vi "Strain_configuration_REV0_2019_02_25.vi"(8 "error in":errorcluster) -> (0 "error out":errorcluster, 3 "task out":refnum<k21>)   [LabVIEW 2017]
uses:
  <vilib>/DAQmx/create/channels.llb/DAQmx Create Channel (AI-Strain-Strain Gage).vi
  <resource>/objmgr/daqmx.rc
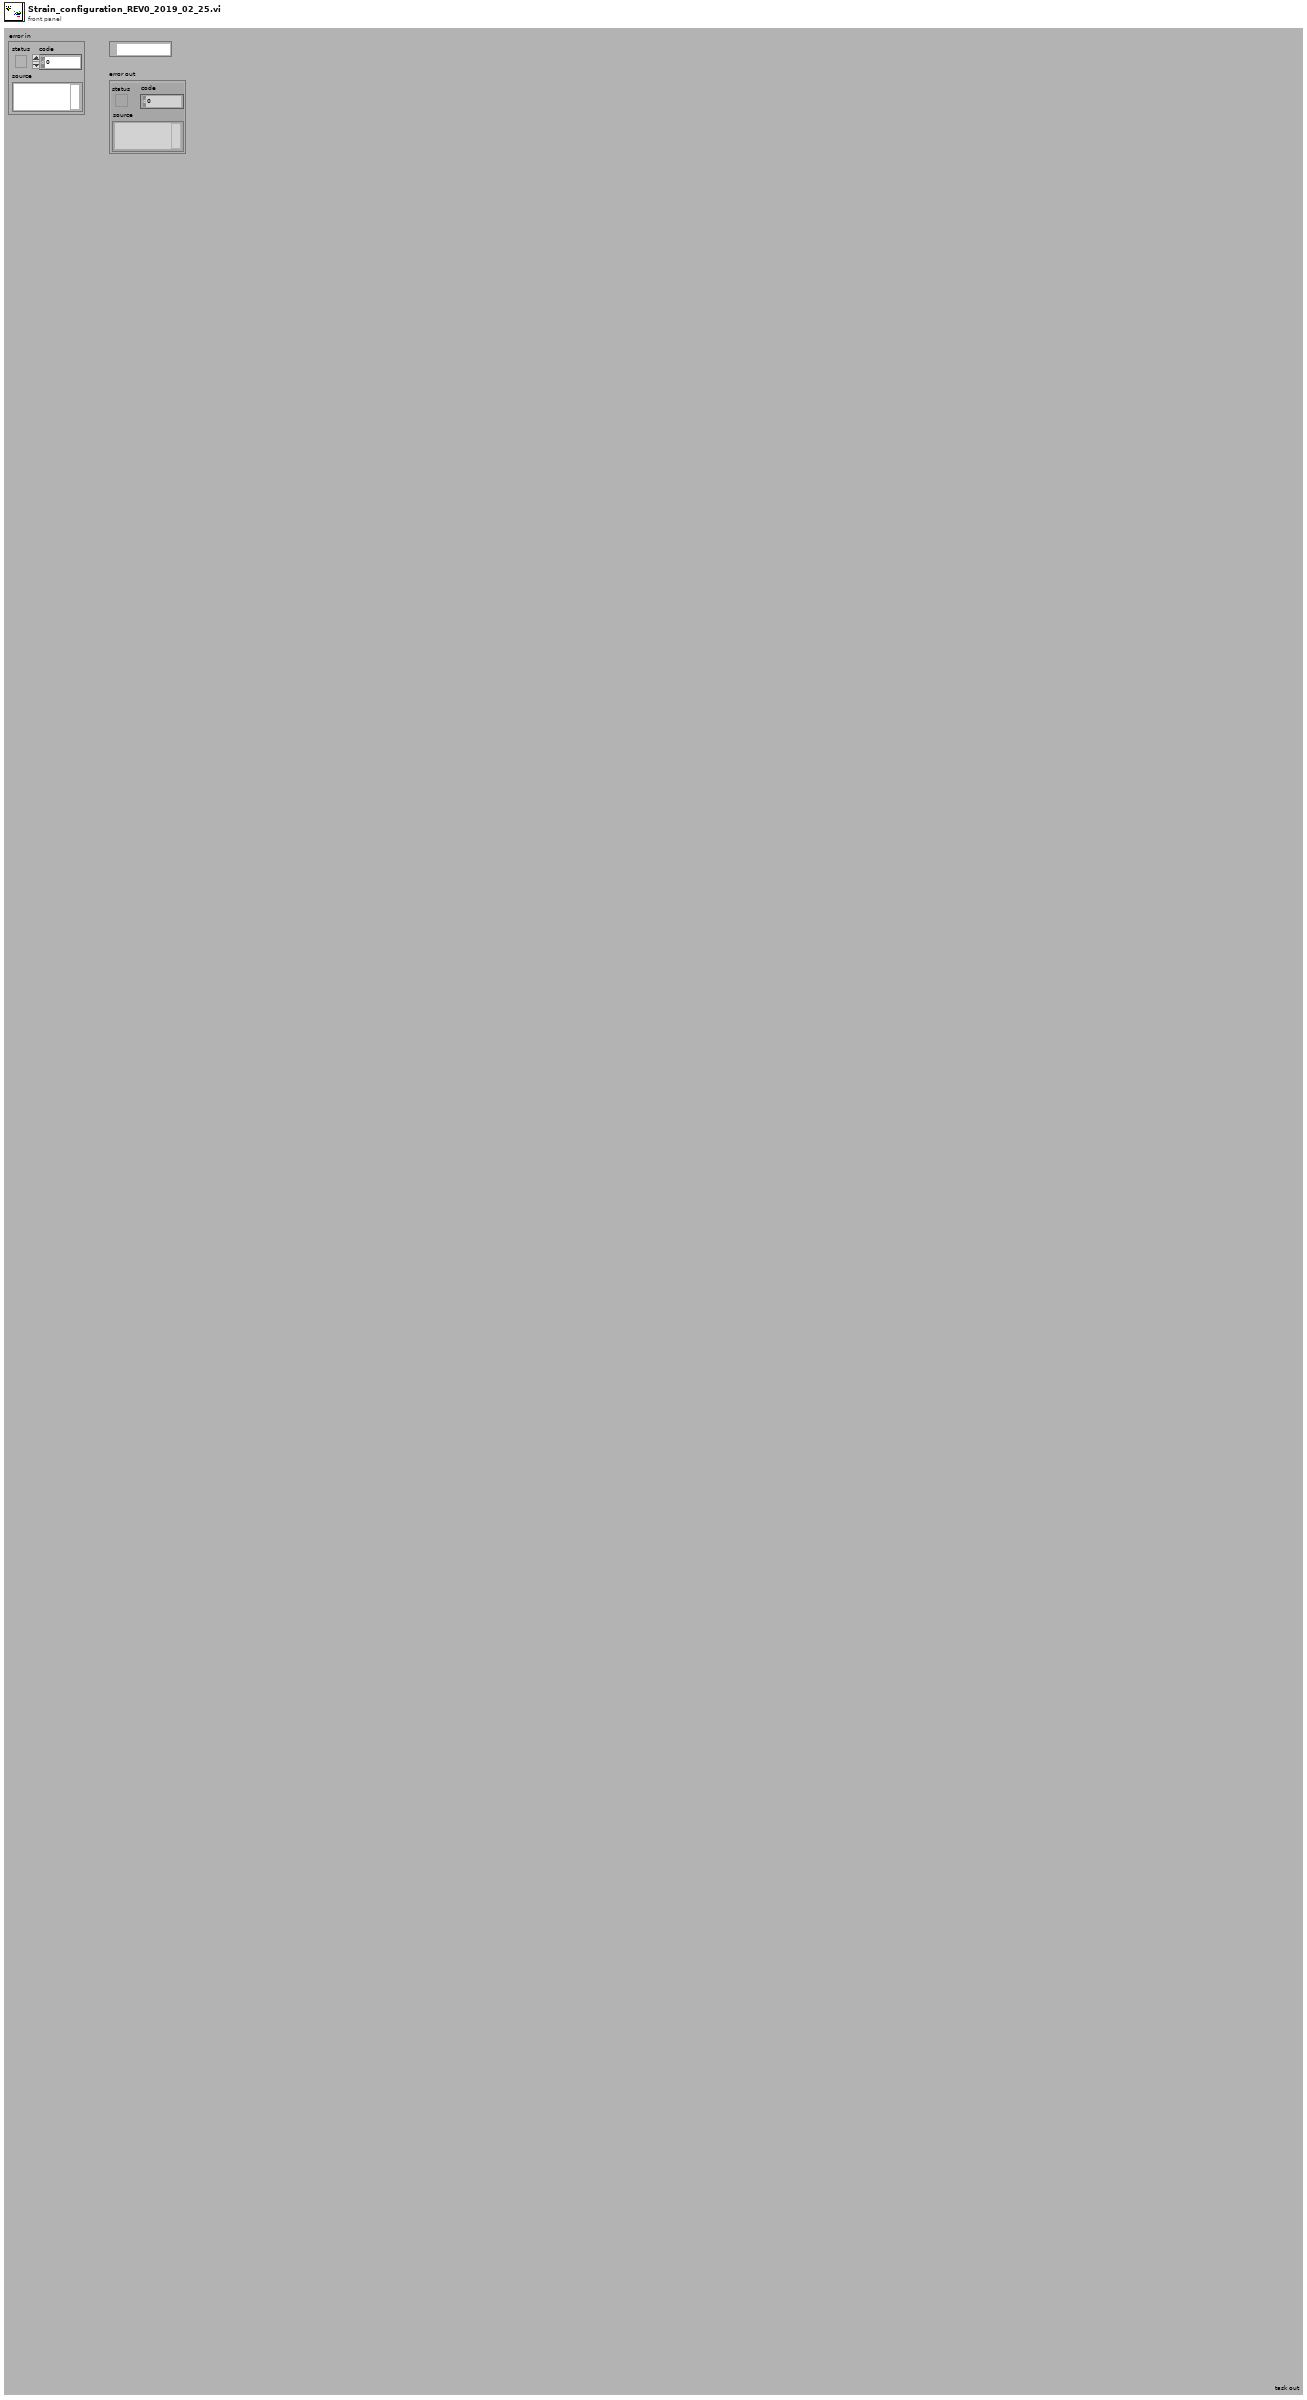
[diagram p1: front panel]
types:
  T1 = cluster{"strain configuration":i32, "lead resistance":dbl, "initial bridge voltage":dbl, "excitation source":i32, "excitation value":dbl}
  T2 = cluster{"gage factor":dbl, "nominal gage resistance":dbl, "poisson ratio":dbl}
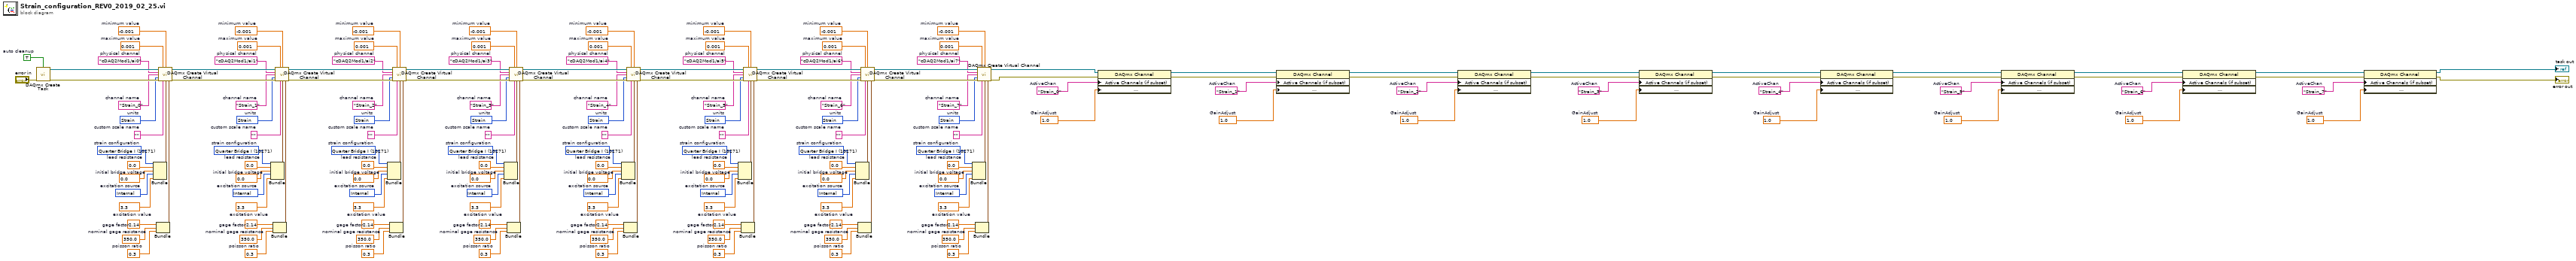
[diagram p0: block diagram]
diagram:
  w3 = 1.0  # GainAdjust
  w5 = "Strain_7"  # ActiveChan
  w6 = 1.0  # GainAdjust
  w9 = "Strain_6"  # ActiveChan
  w10 = 1.0  # GainAdjust
  w13 = "Strain_5"  # ActiveChan
  w14 = 1.0  # GainAdjust
  w17 = "Strain_4"  # ActiveChan
  w18 = 1.0  # GainAdjust
  w21 = "Strain_3"  # ActiveChan
  w22 = 1.0  # GainAdjust
  w25 = "Strain_2"  # ActiveChan
  w26 = 1.0  # GainAdjust
  w29 = "Strain_1"  # ActiveChan
  w30 = 1.0  # GainAdjust
  w33 = "Strain_0"  # ActiveChan
  w38 = 0.0  # lead resistance
  w41 = 0.3  # poisson ratio
  w37 = 0.0  # initial bridge voltage
  w42 = 350.0  # nominal gage resistance
  w40 = 2.14  # gage factor
  w35 = 3.3  # excitation value
  w36 = 10200 items=["Internal"=10200, "External"=10167, "None"=10230]  # excitation source
  w39 = 10271 items=["Full Bridge I"=10183, "Full Bridge II"=10184, "Full Bridge III"=10185, "Half Bridge I"=10188, "Half Bridge II"=10189, "Quarter Bridge I"=10271, "Quarter Bridge II"=10272]  # strain configuration
  w44 = 10299 items=["Strain"=10299, "From Custom Scale"=10065]  # units
  w45 = "Strain_7"  # channel name
  w47 = ""  # custom scale name
  w48 = -0.001  # minimum value
  w49 = 0.001  # maximum value
  w50 = "cDAQ2Mod1/ai7"  # physical channel
  w56 = 0.0  # lead resistance
  w59 = 0.3  # poisson ratio
  w55 = 0.0  # initial bridge voltage
  w60 = 350.0  # nominal gage resistance
  w58 = 2.14  # gage factor
  w53 = 3.3  # excitation value
  w54 = 10200 items=["Internal"=10200, "External"=10167, "None"=10230]  # excitation source
  w57 = 10271 items=["Full Bridge I"=10183, "Full Bridge II"=10184, "Full Bridge III"=10185, "Half Bridge I"=10188, "Half Bridge II"=10189, "Quarter Bridge I"=10271, "Quarter Bridge II"=10272]  # strain configuration
  w62 = 10299 items=["Strain"=10299, "From Custom Scale"=10065]  # units
  w63 = "Strain_6"  # channel name
  w65 = ""  # custom scale name
  w66 = -0.001  # minimum value
  w67 = 0.001  # maximum value
  w68 = "cDAQ2Mod1/ai6"  # physical channel
  w74 = 0.0  # lead resistance
  w77 = 0.3  # poisson ratio
  w73 = 0.0  # initial bridge voltage
  w78 = 350.0  # nominal gage resistance
  w76 = 2.14  # gage factor
  w71 = 3.3  # excitation value
  w72 = 10200 items=["Internal"=10200, "External"=10167, "None"=10230]  # excitation source
  w75 = 10271 items=["Full Bridge I"=10183, "Full Bridge II"=10184, "Full Bridge III"=10185, "Half Bridge I"=10188, "Half Bridge II"=10189, "Quarter Bridge I"=10271, "Quarter Bridge II"=10272]  # strain configuration
  w80 = 10299 items=["Strain"=10299, "From Custom Scale"=10065]  # units
  w81 = "Strain_5"  # channel name
  w83 = ""  # custom scale name
  w84 = -0.001  # minimum value
  w85 = 0.001  # maximum value
  w86 = "cDAQ2Mod1/ai5"  # physical channel
  w92 = 0.0  # lead resistance
  w95 = 0.3  # poisson ratio
  w91 = 0.0  # initial bridge voltage
  w96 = 350.0  # nominal gage resistance
  w94 = 2.14  # gage factor
  w89 = 3.3  # excitation value
  w90 = 10200 items=["Internal"=10200, "External"=10167, "None"=10230]  # excitation source
  w93 = 10271 items=["Full Bridge I"=10183, "Full Bridge II"=10184, "Full Bridge III"=10185, "Half Bridge I"=10188, "Half Bridge II"=10189, "Quarter Bridge I"=10271, "Quarter Bridge II"=10272]  # strain configuration
  w98 = 10299 items=["Strain"=10299, "From Custom Scale"=10065]  # units
  w99 = "Strain_4"  # channel name
  w101 = ""  # custom scale name
  w102 = -0.001  # minimum value
  w103 = 0.001  # maximum value
  w104 = "cDAQ2Mod1/ai4"  # physical channel
  w110 = 0.0  # lead resistance
  w113 = 0.3  # poisson ratio
  w109 = 0.0  # initial bridge voltage
  w114 = 350.0  # nominal gage resistance
  w112 = 2.14  # gage factor
  w107 = 3.3  # excitation value
  w108 = 10200 items=["Internal"=10200, "External"=10167, "None"=10230]  # excitation source
  w111 = 10271 items=["Full Bridge I"=10183, "Full Bridge II"=10184, "Full Bridge III"=10185, "Half Bridge I"=10188, "Half Bridge II"=10189, "Quarter Bridge I"=10271, "Quarter Bridge II"=10272]  # strain configuration
  w116 = 10299 items=["Strain"=10299, "From Custom Scale"=10065]  # units
  w117 = "Strain_3"  # channel name
  w119 = ""  # custom scale name
  w120 = -0.001  # minimum value
  w121 = 0.001  # maximum value
  w122 = "cDAQ2Mod1/ai3"  # physical channel
  w128 = 0.0  # lead resistance
  w131 = 0.3  # poisson ratio
  w127 = 0.0  # initial bridge voltage
  w132 = 350.0  # nominal gage resistance
  w130 = 2.14  # gage factor
  w125 = 3.3  # excitation value
  w126 = 10200 items=["Internal"=10200, "External"=10167, "None"=10230]  # excitation source
  w129 = 10271 items=["Full Bridge I"=10183, "Full Bridge II"=10184, "Full Bridge III"=10185, "Half Bridge I"=10188, "Half Bridge II"=10189, "Quarter Bridge I"=10271, "Quarter Bridge II"=10272]  # strain configuration
  w134 = 10299 items=["Strain"=10299, "From Custom Scale"=10065]  # units
  w135 = "Strain_2"  # channel name
  w137 = ""  # custom scale name
  w138 = -0.001  # minimum value
  w139 = 0.001  # maximum value
  w140 = "cDAQ2Mod1/ai2"  # physical channel
  w146 = 0.0  # lead resistance
  w149 = 0.3  # poisson ratio
  w145 = 0.0  # initial bridge voltage
  w150 = 350.0  # nominal gage resistance
  w148 = 2.14  # gage factor
  w143 = 3.3  # excitation value
  w144 = 10200 items=["Internal"=10200, "External"=10167, "None"=10230]  # excitation source
  w147 = 10271 items=["Full Bridge I"=10183, "Full Bridge II"=10184, "Full Bridge III"=10185, "Half Bridge I"=10188, "Half Bridge II"=10189, "Quarter Bridge I"=10271, "Quarter Bridge II"=10272]  # strain configuration
  w152 = 10299 items=["Strain"=10299, "From Custom Scale"=10065]  # units
  w153 = "Strain_1"  # channel name
  w155 = ""  # custom scale name
  w156 = -0.001  # minimum value
  w157 = 0.001  # maximum value
  w158 = "cDAQ2Mod1/ai1"  # physical channel
  w164 = 0.0  # lead resistance
  w167 = 0.3  # poisson ratio
  w163 = 0.0  # initial bridge voltage
  w168 = 350.0  # nominal gage resistance
  w166 = 2.14  # gage factor
  w161 = 3.3  # excitation value
  w162 = 10200 items=["Internal"=10200, "External"=10167, "None"=10230]  # excitation source
  w165 = 10271 items=["Full Bridge I"=10183, "Full Bridge II"=10184, "Full Bridge III"=10185, "Half Bridge I"=10188, "Half Bridge II"=10189, "Quarter Bridge I"=10271, "Quarter Bridge II"=10272]  # strain configuration
  w170 = 10299 items=["Strain"=10299, "From Custom Scale"=10065]  # units
  w171 = "Strain_0"  # channel name
  w173 = ""  # custom scale name
  w174 = -0.001  # minimum value
  w175 = 0.001  # maximum value
  w176 = "cDAQ2Mod1/ai0"  # physical channel
  w178 = TRUE  # auto cleanup
  n1 = call <vilib>:"DAQmx Create Task.vi"("auto cleanup"=w178, "error in"="error in") -> ("task out"=w177:refnum<k21>, "error out"=w179:errorcluster)  [unwired: 12 in]
  n2 = Bundle("strain configuration"=w165, "lead resistance"=w164, "initial bridge voltage"=w163, "excitation source"=w162, "excitation value"=w161) -> (w160:T1)  [unwired: 1 in]
  n3 = Bundle("gage factor"=w166, "nominal gage resistance"=w168, "poisson ratio"=w167) -> (w169:T2)  [unwired: 1 in]
  n4 = call-poly <vilib>:"DAQmx Create Virtual Channel.vi"("task in"=w177, "maximum value"=w175, "minimum value"=w174, "physical channels"=w176, "name to assign"=w171, "units"=w170, "error in"=w179, "custom scale name"=w173, "bridge information"=w160, "strain gage information"=w169) -> ("task out"=w159:refnum<k21>, "error out"=w172:errorcluster)  [unwired: 4 in]
  n5 = Bundle("strain configuration"=w147, "lead resistance"=w146, "initial bridge voltage"=w145, "excitation source"=w144, "excitation value"=w143) -> (w142:T1)  [unwired: 1 in]
  n6 = Bundle("gage factor"=w148, "nominal gage resistance"=w150, "poisson ratio"=w149) -> (w151:T2)  [unwired: 1 in]
  n7 = call-poly <vilib>:"DAQmx Create Virtual Channel.vi"("task in"=w159, "maximum value"=w157, "minimum value"=w156, "physical channels"=w158, "name to assign"=w153, "units"=w152, "error in"=w172, "custom scale name"=w155, "bridge information"=w142, "strain gage information"=w151) -> ("task out"=w141:refnum<k21>, "error out"=w154:errorcluster)  [unwired: 4 in]
  n8 = Bundle("strain configuration"=w129, "lead resistance"=w128, "initial bridge voltage"=w127, "excitation source"=w126, "excitation value"=w125) -> (w124:T1)  [unwired: 1 in]
  n9 = Bundle("gage factor"=w130, "nominal gage resistance"=w132, "poisson ratio"=w131) -> (w133:T2)  [unwired: 1 in]
  n10 = call-poly <vilib>:"DAQmx Create Virtual Channel.vi"("task in"=w141, "maximum value"=w139, "minimum value"=w138, "physical channels"=w140, "name to assign"=w135, "units"=w134, "error in"=w154, "custom scale name"=w137, "bridge information"=w124, "strain gage information"=w133) -> ("task out"=w123:refnum<k21>, "error out"=w136:errorcluster)  [unwired: 4 in]
  n11 = Bundle("strain configuration"=w111, "lead resistance"=w110, "initial bridge voltage"=w109, "excitation source"=w108, "excitation value"=w107) -> (w106:T1)  [unwired: 1 in]
  n12 = Bundle("gage factor"=w112, "nominal gage resistance"=w114, "poisson ratio"=w113) -> (w115:T2)  [unwired: 1 in]
  n13 = call-poly <vilib>:"DAQmx Create Virtual Channel.vi"("task in"=w123, "maximum value"=w121, "minimum value"=w120, "physical channels"=w122, "name to assign"=w117, "units"=w116, "error in"=w136, "custom scale name"=w119, "bridge information"=w106, "strain gage information"=w115) -> ("task out"=w105:refnum<k21>, "error out"=w118:errorcluster)  [unwired: 4 in]
  n14 = Bundle("strain configuration"=w93, "lead resistance"=w92, "initial bridge voltage"=w91, "excitation source"=w90, "excitation value"=w89) -> (w88:T1)  [unwired: 1 in]
  n15 = Bundle("gage factor"=w94, "nominal gage resistance"=w96, "poisson ratio"=w95) -> (w97:T2)  [unwired: 1 in]
  n16 = call-poly <vilib>:"DAQmx Create Virtual Channel.vi"("task in"=w105, "maximum value"=w103, "minimum value"=w102, "physical channels"=w104, "name to assign"=w99, "units"=w98, "error in"=w118, "custom scale name"=w101, "bridge information"=w88, "strain gage information"=w97) -> ("task out"=w87:refnum<k21>, "error out"=w100:errorcluster)  [unwired: 4 in]
  n17 = Bundle("strain configuration"=w75, "lead resistance"=w74, "initial bridge voltage"=w73, "excitation source"=w72, "excitation value"=w71) -> (w70:T1)  [unwired: 1 in]
  n18 = Bundle("gage factor"=w76, "nominal gage resistance"=w78, "poisson ratio"=w77) -> (w79:T2)  [unwired: 1 in]
  n19 = call-poly <vilib>:"DAQmx Create Virtual Channel.vi"("task in"=w87, "maximum value"=w85, "minimum value"=w84, "physical channels"=w86, "name to assign"=w81, "units"=w80, "error in"=w100, "custom scale name"=w83, "bridge information"=w70, "strain gage information"=w79) -> ("task out"=w69:refnum<k21>, "error out"=w82:errorcluster)  [unwired: 4 in]
  n20 = Bundle("strain configuration"=w57, "lead resistance"=w56, "initial bridge voltage"=w55, "excitation source"=w54, "excitation value"=w53) -> (w52:T1)  [unwired: 1 in]
  n21 = Bundle("gage factor"=w58, "nominal gage resistance"=w60, "poisson ratio"=w59) -> (w61:T2)  [unwired: 1 in]
  n22 = call-poly <vilib>:"DAQmx Create Virtual Channel.vi"("task in"=w69, "maximum value"=w67, "minimum value"=w66, "physical channels"=w68, "name to assign"=w63, "units"=w62, "error in"=w82, "custom scale name"=w65, "bridge information"=w52, "strain gage information"=w61) -> ("task out"=w51:refnum<k21>, "error out"=w64:errorcluster)  [unwired: 4 in]
  n23 = Bundle("strain configuration"=w39, "lead resistance"=w38, "initial bridge voltage"=w37, "excitation source"=w36, "excitation value"=w35) -> (w34:T1)  [unwired: 1 in]
  n24 = Bundle("gage factor"=w40, "nominal gage resistance"=w42, "poisson ratio"=w41) -> (w43:T2)  [unwired: 1 in]
  n25 = call-poly <vilib>:"DAQmx Create Virtual Channel.vi"("task in"=w51, "maximum value"=w49, "minimum value"=w48, "physical channels"=w50, "name to assign"=w45, "units"=w44, "error in"=w64, "custom scale name"=w47, "bridge information"=w34, "strain gage information"=w43) -> ("task out"=w32:refnum<k21>, "error out"=w46:errorcluster)  [unwired: 4 in]
  n26 = property class="DAQmx Channel"(reference=w32, error in=w46, "Active Channels (if subset)"=w33, "Analog Input:General Properties:Signal Conditioning:Bridge:Shunt Cal:Gain Adjustment"=w30) -> (reference out=w28:refnum<k21>, error out=w31:errorcluster)
  n27 = property class="DAQmx Channel"(reference=w28, error in=w31, "Active Channels (if subset)"=w29, "Analog Input:General Properties:Signal Conditioning:Bridge:Shunt Cal:Gain Adjustment"=w26) -> (reference out=w24:refnum<k21>, error out=w27:errorcluster)
  n28 = property class="DAQmx Channel"(reference=w24, error in=w27, "Active Channels (if subset)"=w25, "Analog Input:General Properties:Signal Conditioning:Bridge:Shunt Cal:Gain Adjustment"=w22) -> (reference out=w20:refnum<k21>, error out=w23:errorcluster)
  n29 = property class="DAQmx Channel"(reference=w20, error in=w23, "Active Channels (if subset)"=w21, "Analog Input:General Properties:Signal Conditioning:Bridge:Shunt Cal:Gain Adjustment"=w18) -> (reference out=w16:refnum<k21>, error out=w19:errorcluster)
  n30 = property class="DAQmx Channel"(reference=w16, error in=w19, "Active Channels (if subset)"=w17, "Analog Input:General Properties:Signal Conditioning:Bridge:Shunt Cal:Gain Adjustment"=w14) -> (reference out=w12:refnum<k21>, error out=w15:errorcluster)
  n31 = property class="DAQmx Channel"(reference=w12, error in=w15, "Active Channels (if subset)"=w13, "Analog Input:General Properties:Signal Conditioning:Bridge:Shunt Cal:Gain Adjustment"=w10) -> (reference out=w8:refnum<k21>, error out=w11:errorcluster)
  n32 = property class="DAQmx Channel"(reference=w8, error in=w11, "Active Channels (if subset)"=w9, "Analog Input:General Properties:Signal Conditioning:Bridge:Shunt Cal:Gain Adjustment"=w6) -> (reference out=w4:refnum<k21>, error out=w7:errorcluster)
  n33 = property class="DAQmx Channel"(reference=w4, error in=w7, "Active Channels (if subset)"=w5, "Analog Input:General Properties:Signal Conditioning:Bridge:Shunt Cal:Gain Adjustment"=w3) -> (reference out=→"task out":refnum<k21>, error out=→"error out":errorcluster)
